vi "Main.vi"(11 "Module Admin":refnum<class "Delacor_lib_QMH_Cloneable Module Admin.lvclass">) -> ()   [LabVIEW 2019, in "Adquisicion2.lvlib"]
doc: "This template is based off of the Queued Message Handler design pattern and the Queued Message Handler project template that ships with LabVIEW.\n\nThe main difference is that the queue is private to this module and communication between modules is performed via Broadcast and Request events.\n\nRequest events are wrapped in public API methods and are handled in the Event Handling Loop (EHL) of this VI. Any module can register for Broadcast events sent by this module. The EHL generates messages based on user interface actions.\n\nThe Message Handling Loop (MHL) processes messages generated by the EHL, or by other messages. The messages are string values, so new messages can be added easily to the Message Cases case structure in the MHL. Each message cluster can also provide an optional value for Message Data, which is a variant that can be converted to whatever message-specific data is required.\n_____\nBased on Delacor QMH Project Template 5.0.0.82."
uses:
  Adquisicion2.lvlib
  <vilib>/Delacor/Delacor QMH/Libraries/Cloneable Module Admin_class/Delacor_lib_QMH_Cloneable Module Admin.lvclass
  C:/Program Files/National Instruments/LabVIEW 2019/vi.lib/Delacor/Delacor QMH/Libraries/Module Admin_class/Delacor_lib_QMH_Module Admin.lvclass
  Module Data--cluster.ctl
  <vilib>/Delacor/Delacor QMH/Libraries/Message Queue_class/Delacor_lib_QMH_Message Queue.lvclass/Delacor_lib_QMH_Message Queue.ctl
  <vilib>/Delacor/Delacor QMH/Libraries/Cloneable Module Admin_class/Delacor_lib_QMH_Cloneable Module Admin.lvclass/Delacor_lib_QMH_Cloneable Module Admin.ctl
  Stop Argument--cluster.ctl
  <vilib>/Delacor/Delacor QMH/Libraries/Module Admin_class/Delacor_lib_QMH_Module Admin.lvclass/Delacor_lib_QMH_Module Admin.ctl
  <vilib>/Utility/miscctls.llb/LVPointTypeDef.ctl
  <vilib>/Delacor/Delacor QMH/Libraries/Message Queue_class/Delacor_lib_QMH_Enqueue Message (Single).vi
  <vilib>/Delacor/Delacor QMH/Libraries/Cloneable Module Admin_class/Delacor_lib_QMH_Get Module ID.vi
  <vilib>/Delacor/Delacor QMH/Libraries/Module Admin_class/Delacor_lib_QMH_Get External Launch.vi
  <vilib>/Utility/error.llb/Error Cluster From Error Code.vi
  <vilib>/ErrorRing/Error Ring.xnode
  <vilib>/Delacor/Delacor QMH/Libraries/Message Queue_class/Delacor_lib_QMH_Message Queue.lvclass
panel:
  in  "Simulate MHL Error":bool
  in  "Simulate EHL Error":bool
  out "error out":errorcluster
  out "Status":string
  # "Other QMH Modules communicate with this Module via its Public API (wrappers for its Request Events).\n\nThis Module communicates with other Modules via its Broadcast Events.\nAny module that wants to get these messages, just registers for this module's Broadcast events."
  # "This template is for the Delacor Modified Queued Message Handler design pattern.\n\nSee the block diagram for more information on how to use this template."
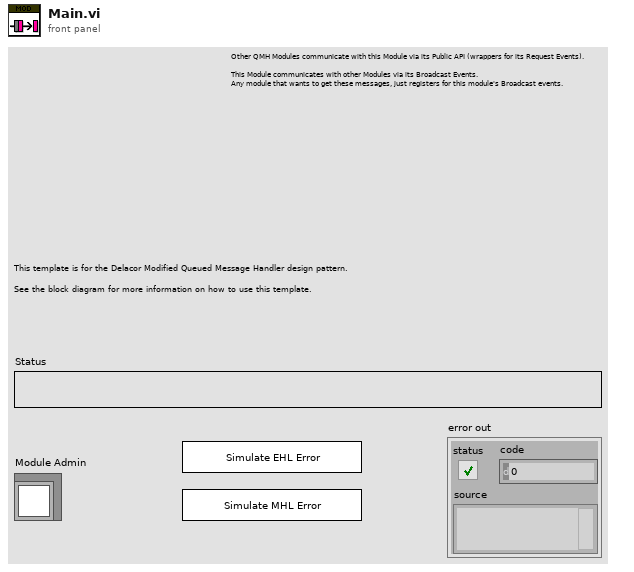
[diagram p1: front panel]
types:
  T1 = typedef "Adquisicion2.lvlib/Request Events--cluster.ctl" = cluster{"Stop Module":refnum<user-event>, "Show Panel":refnum<user-event>, "Hide Panel":refnum<user-event>, "Show Diagram":refnum<user-event>, "Get Module Execution Status":refnum<user-event>}
  T2 = typedef "Adquisicion2.lvlib/Module Data--cluster.ctl" = cluster{"Status":string}
  T3 = enum32{"invalid lock state", "Not Locked", "Locked (No Password)", "Password-protected"}
  T4 = typedef "Adquisicion2.lvlib/Stop Argument--cluster.ctl" = cluster{"Module ID":i32, "Origin":string, "Exit via Stop Module Req?":bool, "Wait for Module to stop?":bool}
  T5 = typedef "LVPointTypeDef.ctl" = cluster{"Horizontal":i16, "Vertical":i16}
  T6 = enum32{"Invalid", "Standard", "Closed", "Hidden", "Minimized", "Maximized"}
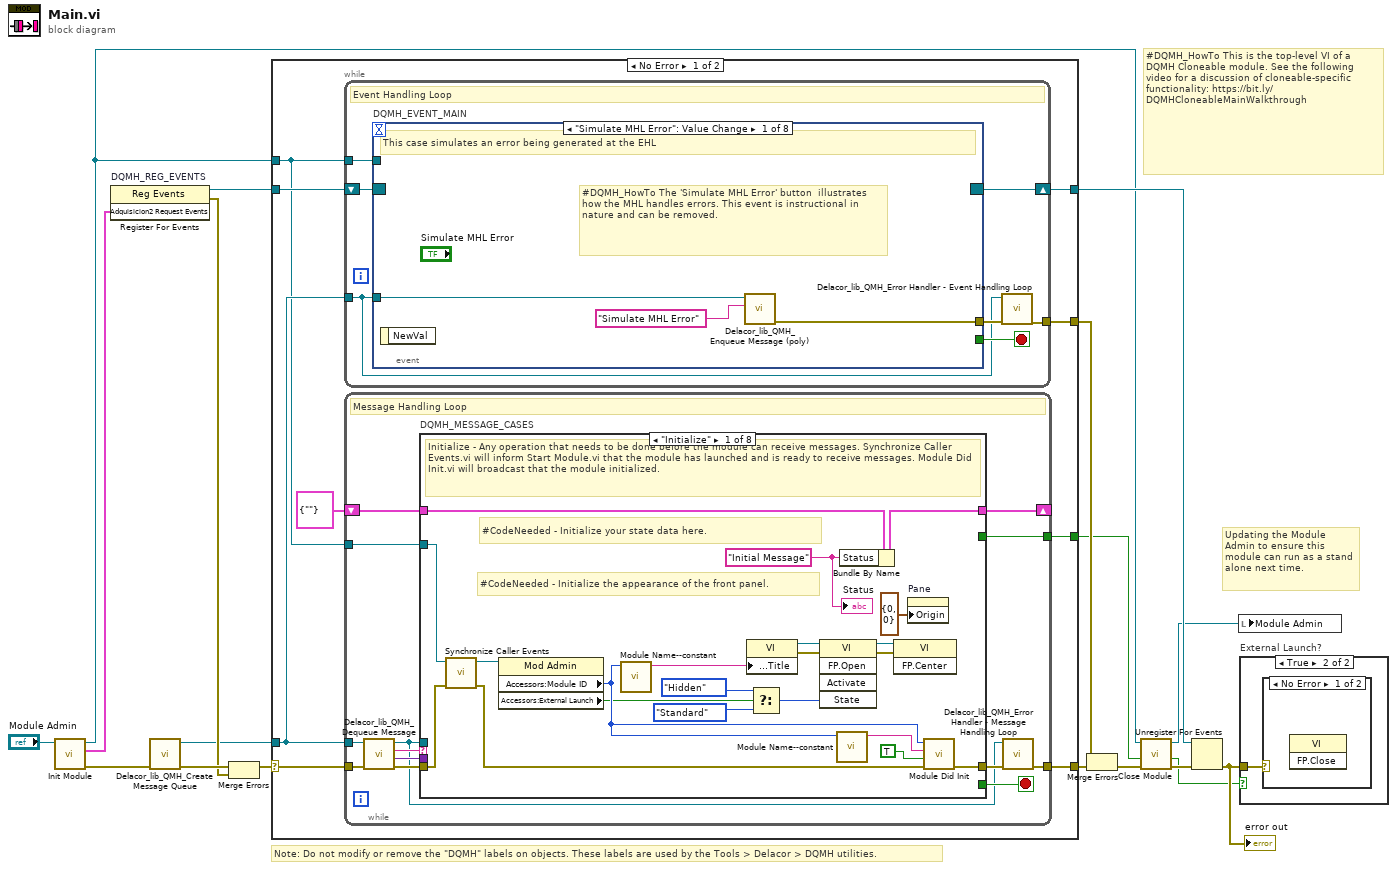
[diagram p0: block diagram]
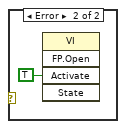
[diagram p3: hidden frame]
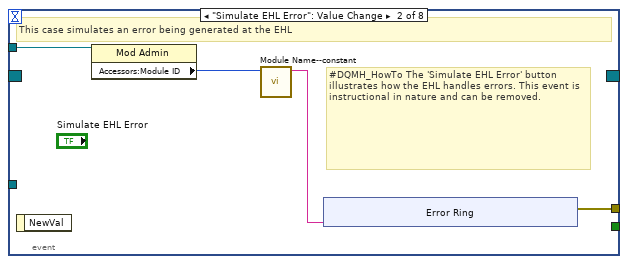
[diagram p4: hidden frame]
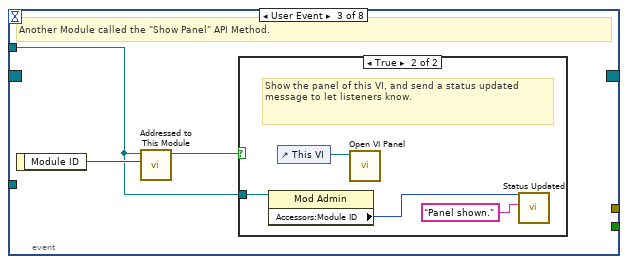
[diagram p5: hidden frame]
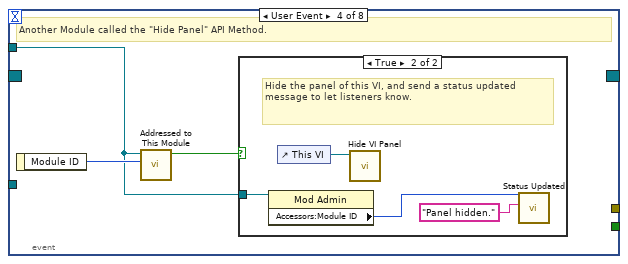
[diagram p7: hidden frame]
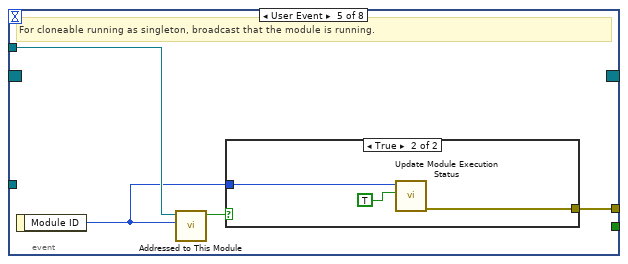
[diagram p9: hidden frame]
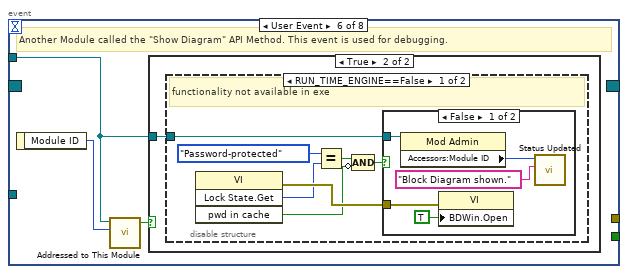
[diagram p11: hidden frame]
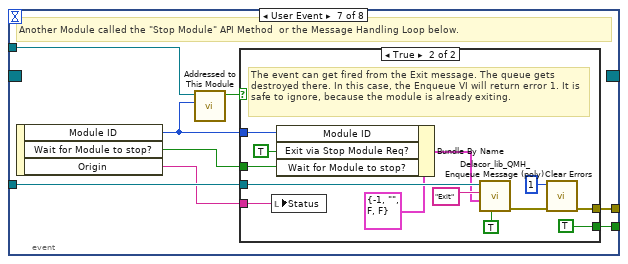
[diagram p15: hidden frame]
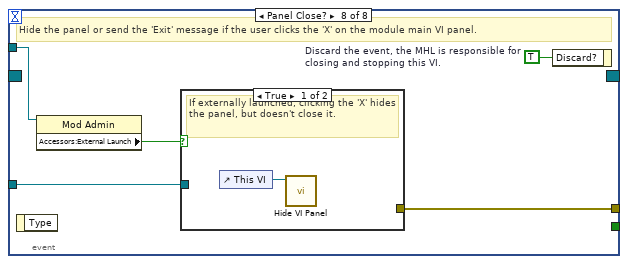
[diagram p17: hidden frame]
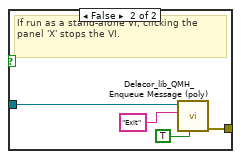
[diagram p18: hidden frame]
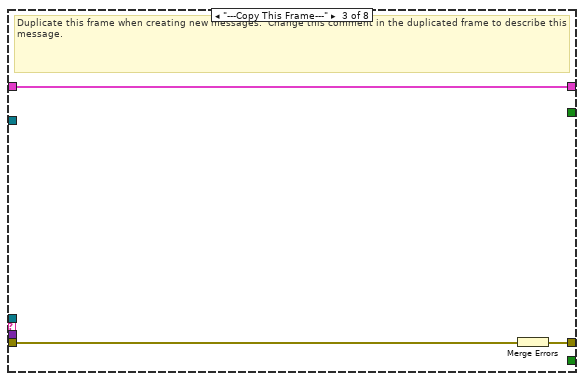
[diagram p20: hidden frame]
diagram:
  # "#DQMH_HowTo This is the top-level VI of a DQMH Cloneable module. See the following video for a discussion of cloneable-specific functionality: https://bit.ly/DQMHCloneableMainWalkthrough"
  # "Note: Do not modify or remove the \"DQMH\" labels on objects. These labels are used by the Tools > Delacor > DQMH utilities."
  # "Updating the Module Admin to ensure this module can run as a stand alone next time."
  n1 = call "Init Module.vi"("Cloneable Module Admin in"="Module Admin") -> ("error out"=w15:errorcluster, "Adquisicion2 Request Events"=w7:T1, "Cloneable Module Admin out"=w4:refnum<class "Delacor_lib_QMH_Cloneable Module Admin.lvclass">)  [unwired: 8 in]
  n2 = register-events "DQMH_REG_EVENTS"(w7) -> (reference out=w8:refnum<event-registration>, error out=w10:errorcluster)  [unwired: 2 in]
  n3 = call <vilib>:"Delacor_lib_QMH_Create Message Queue.vi"("error in (no error)"=w15) -> ("error out"=w12:errorcluster, "Message Queue"=w6:refnum<class "Delacor_lib_QMH_Message Queue.lvclass">)  [unwired: 9 in]
  n4 = Merge Errors(w12, w10) -> (w11:errorcluster)
  n5 = case shown="No Error" w11 {
    selector: w11 -> [w25 w224]
    tunnel: [w27 w223] -> w16
    tunnel: [w24 w231] -> w9
    tunnel: w8 -> [w22 w231]
    tunnel: w6 -> [w21 w222]
    tunnel: [w26 _] -> w17
    tunnel: w4 -> [w20 w227]
    tunnel: [w19 _] -> w2
    frame No Error {
      n6 = while {
        tunnel: w21 -> [w28]
        shift-right: [w31] -> w24
        shift-left: w22 -> [w32]
        tunnel: [w33] -> w26
        tunnel: w20 -> [w29]
        stop <- w30 stop-if-true
        # "Event Handling Loop"
        n7 = event "DQMH_EVENT_MAIN" shown="[0] \"Simulate MHL Error\": Value Change" {
          selector: w32 -> [_ _ _ _ _ _ _ _]
          dyn-events: [_ _ _ _ _ _ _ _] -> w31
          timeout: _ -> [_ _ _ _ _ _ _ _]
          tunnel: [_ _ _ _ _ _ w89 _] -> w30
          tunnel: w28 -> [w36 _ _ _ _ _ w92 w108]
          tunnel: [w37 w41 _ _ w66 _ w93 w111] -> w34
          tunnel: w29 -> [_ w40 w49 w56 w64 w70 w91 w109]
          event "Simulate MHL Error": Value Change {
            # "#DQMH_HowTo The 'Simulate MHL Error' button  illustrates how the MHL handles errors. This event is instructional in nature and can be removed."
            # "This case simulates an error being generated at the EHL"
            n8 = event-data() -> ()  [unwired: 1 in, 1 out]
            n9 = call-poly <vilib>:"Delacor_lib_QMH_Enqueue Message (poly).vi"("Message"="Simulate MHL Error", "Message Queue in"=w36) -> ("error out"=w37:errorcluster)  [unwired: 8 in, 1 out]
          }
          event "Simulate EHL Error": Value Change {
            # "#DQMH_HowTo The 'Simulate EHL Error' button  illustrates how the EHL handles errors. This event is instructional in nature and can be removed."
            # "This case simulates an error being generated at the EHL"
            n10 = event-data() -> ()  [unwired: 1 in, 1 out]
            n11 = property class="Mod Admin"(reference=w40) -> ("Accessors:Module ID"=w39:i32)  [unwired: 1 in, 2 out]
            n12 = call "Module Name--constant.vi"("Module ID"=w39) -> ("Module Name"=w38:string)  [unwired: 10 in]
            n13 = xnode "Error Ring"("parameter 0"=w38) -> ("error out"=w41:errorcluster)
          }
          event User Event {
            # "Another Module called the \"Show Panel\" API Method."
            n14 = event-data() -> ("Module ID"=w50:i32)  [unwired: 1 in]
            n15 = call "Addressed to This Module.vi"("Module ID from Argument"=w50, "Module Admin"=w49) -> ("Addressed to this instance?"=w51:bool)  [unwired: 8 in, 1 out]
            n16 = case shown="True" w51 {
              tunnel: w49 -> [_ w53]
              frame False {
              }
              frame True {
                # "Show the panel of this VI, and send a status updated message to let listeners know."
                n17 = property class="Mod Admin"(reference=w53) -> ("Accessors:Module ID"=w52:i32)  [unwired: 1 in, 2 out]
                n18 = control-ref of="This VI"() -> (w55:refnum<vi>)
                n19 = call "Open VI Panel.vi"("VI"=w55) -> ()  [unwired: 10 in, 1 out]
                n20 = call "Status Updated.vi"("Status"="Panel shown." ("format string"), "Module ID"=w52) -> ()  [unwired: 9 in, 1 out]
              }
            }
          }
          event User Event {
            # "Another Module called the \"Hide Panel\" API Method."
            n21 = event-data() -> ("Module ID"=w57:i32)  [unwired: 1 in]
            n22 = call "Addressed to This Module.vi"("Module ID from Argument"=w57, "Module Admin"=w56) -> ("Addressed to this instance?"=w58:bool)  [unwired: 8 in, 1 out]
            n23 = case shown="True" w58 {
              tunnel: w56 -> [_ w60]
              frame False {
              }
              frame True {
                # "Hide the panel of this VI, and send a status updated message to let listeners know."
                n24 = property class="Mod Admin"(reference=w60) -> ("Accessors:Module ID"=w59:i32)  [unwired: 1 in, 2 out]
                n25 = control-ref of="This VI"() -> (w62:refnum<vi>)
                n26 = call "Hide VI Panel.vi"("VI"=w62) -> ()  [unwired: 10 in, 1 out]
                n27 = call "Status Updated.vi"("Status"="Panel hidden." ("format string"), "Module ID"=w59) -> ()  [unwired: 9 in, 1 out]
              }
            }
          }
          event User Event {
            # "For cloneable running as singleton, broadcast that the module is running."
            n28 = event-data() -> ("Module ID"=w63:i32)  [unwired: 1 in]
            n29 = call "Addressed to This Module.vi"("Module ID from Argument"=w63, "Module Admin"=w64) -> ("Addressed to this instance?"=w65:bool)  [unwired: 8 in, 1 out]
            n30 = case shown="True" w65 {
              tunnel: [_ w69] -> w66
              tunnel: w63 -> [_ w68]
              frame False {
              }
              frame True {
                n31 = call "Update Module Execution Status.vi"("Running?"=TRUE, "Module ID"=w68) -> ("error out"=w69:errorcluster)  [unwired: 9 in]
              }
            }
          }
          event User Event {
            # "Another Module called the \"Show Diagram\" API Method. This event is used for debugging."
            n32 = event-data() -> ("Module ID"=w71:i32)  [unwired: 1 in]
            n33 = call "Addressed to This Module.vi"("Module ID from Argument"=w71, "Module Admin"=w70) -> ("Addressed to this instance?"=w72:bool)  [unwired: 8 in, 1 out]
            n34 = case shown="True" w72 {
              tunnel: w70 -> [_ w73]
              frame False {
              }
              frame True {
                n35 = disable-structure shown="RUN_TIME_ENGINE==False" {
                  disable-tunnel: w73 -> [w74 _]
                  frame condition #0 (active) {
                    # "functionality not available in exe"
                    n36 = invoke class="VI" method="Lock State.Get"() -> (error out=w80:errorcluster, "Get Lock State"=w79:T3, "pwd in cache"=w76:bool)  [unwired: 4 in, 1 out]
                    n37 = Equal?(x=T3."Password-protected", y=w79) -> (x = y?=w77:bool)
                    n38 = Compound Arithmetic op=AND(w77, invert w76) -> (w75:bool)
                    n39 = case shown="False" w75 {
                      tunnel: w80 -> [w85 _]
                      tunnel: w74 -> [w82 _]
                      frame False {
                        n40 = property class="Mod Admin"(reference=w82) -> ("Accessors:Module ID"=w81:i32)  [unwired: 1 in, 2 out]
                        n41 = property class="VI"(error in=w85, "BDWin.Open"=TRUE ("Block Diagram Window:Open")) -> ()  [unwired: 1 in, 2 out]
                        n42 = call "Status Updated.vi"("Status"="Block Diagram shown." ("format string"), "Module ID"=w81) -> ()  [unwired: 9 in, 1 out]
                      }
                      frame True {
                        # "Password-protected VI, and the password is not in the cache. Do not show the diagram."
                      }
                    }
                  }
                  frame condition #1 {
                  }
                }
              }
            }
          }
          event User Event {
            # "Another Module called the \"Stop Module\" API Method  or the Message Handling Loop below."
            n43 = event-data() -> ("Module ID"=w87:i32, "Wait for Module to stop?"=w88:bool, "Origin"=w86:string)  [unwired: 1 in]
            n44 = call "Addressed to This Module.vi"("Module ID from Argument"=w87, "Module Admin"=w91) -> ("Addressed to this instance?"=w90:bool)  [unwired: 8 in, 1 out]
            n45 = case shown="True" w90 {
              tunnel: [_ w105] -> w93
              tunnel: w92 -> [_ w101]
              tunnel: [_ TRUE] -> w89
              tunnel: w88 -> [_ w96]
              tunnel: w87 -> [_ w98]
              tunnel: w86 -> [_ w94]
              frame False {
              }
              frame True {
                # "The event can get fired from the Exit message. The queue gets destroyed there. In this case, the Enqueue VI will return error 1. It is safe to ignore, because the module is already exiting."
                n46 = local write "Status"(w94) -> ()
                n47 = Bundle By Name(cluster=T4 {"Module ID"=-1, "Origin"="", "Exit via Stop Module Req?"=FALSE, "Wait for Module to stop?"=FALSE} ("Stop Argument"), "Module ID"=w98, "Exit via Stop Module Req?"=TRUE, "Wait for Module to stop?"=w96) -> (w95:T4)
                n48 = call-poly <vilib>:"Delacor_lib_QMH_Enqueue Message (poly).vi"("Priority Message? (F)"=TRUE, "Message Data"=w95, "Message"="Exit", "Message Queue in"=w101) -> ("error out"=w106:errorcluster)  [unwired: 6 in, 1 out]
                n49 = call <vilib>:"Clear Errors.vi"("error in (no error)"=w106, "specific error code to clear (0: all)"=1) -> ("error out"=w105:errorcluster)  [unwired: 4 in, 1 out]
              }
            }
          }
          event Panel Close? {
            w110 = TRUE  # Discard the event, the MHL is responsible for closing and stopping this VI.
            # "Hide the panel or send the 'Exit' message if the user clicks the 'X' on the module main VI panel."
            n50 = event-data() -> ()  [unwired: 1 in, 1 out]
            n51 = property class="Mod Admin"(reference=w109) -> ("Accessors:External Launch"=w107:bool)  [unwired: 1 in, 2 out]
            n52 = case shown="True" w107 {
              tunnel: w108 -> [_ w115]
              tunnel: [_ w116] -> w111
              frame True {
                # "If externally launched, clicking the 'X' hides the panel, but doesn't close it."
                n53 = control-ref of="This VI"() -> (w112:refnum<vi>)
                n54 = call "Hide VI Panel.vi"("VI"=w112) -> ()  [unwired: 10 in, 1 out]
              }
              frame False {
                # "If run as a stand-alone VI, clicking the panel 'X' stops the VI."
                n55 = call-poly <vilib>:"Delacor_lib_QMH_Enqueue Message (poly).vi"("Priority Message? (F)"=TRUE, "Message"="Exit", "Message Queue in"=w115) -> ("error out"=w116:errorcluster)  [unwired: 7 in, 1 out]
              }
            }
            n56 = event-data("Discard?"=w110) -> ()  [unwired: 1 in, 1 out]
          }
        }
        n57 = call-dynamic "Delacor_lib_QMH_Error Handler - Event Handling Loop.vi"("error in (no error)"=w34, "Message Queue in"=w28) -> ("dup error in"=w33:errorcluster)  [unwired: 8 in, 1 out]
      }
      n58 = while {
        tunnel: w21 -> [w120]
        shift-right: [w124] -> _
        shift-left: T2 {"Status"=""} ("Data Cluster") -> [w125]
        tunnel: w25 -> [w128]
        tunnel: [w126] -> w27
        tunnel: w20 -> [w118]
        tunnel: [w117] -> w19
        stop <- w123 stop-if-true
        # "Message Handling Loop"
        n59 = call-dynamic "Delacor_lib_QMH_Dequeue Message.vi"("error in (no error)"=w128, "Message Queue in"=w120) -> ("error out"=w127:errorcluster, "Message Data"=w121:variant, "Message"=w122:string, "Message Queue out"=w119:refnum<class "Delacor_lib_QMH_Message Queue.lvclass">)  [unwired: 6 in]
        n60 = case "DQMH_MESSAGE_CASES" shown="\"Initialize\"" w122 {
          selector: w122 -> [_ _ _ _ _ _ _ w209]
          tunnel: w119 -> [_ _ _ _ w160 _ w199 _]
          tunnel: w127 -> [w148 w152 w155 w157 w169 w182 w205 w211]
          tunnel: [w146 w152 w154 w157 w165 w181 w202 w212] -> w129
          tunnel: w125 -> [w139 w151 w153 w156 w164 w179 w198 w210]
          tunnel: [w138 w151 w153 w156 w164 w179 w198 w210] -> w124
          tunnel: [_ _ _ _ _ _ w197 _] -> w123
          tunnel: w121 -> [_ _ _ _ w163 _ w195 _]
          tunnel: w118 -> [w133 _ _ _ w162 w177 w191 w207]
          tunnel: [_ _ _ _ _ _ w193 _] -> w117
          frame "Initialize" {
            w130 = "Initial Message" ("Initial Message")
            # "#CodeNeeded - Initialize the appearance of the front panel."
            # "#CodeNeeded - Initialize your state data here."
            # "Initialize - Any operation that needs to be done before the module can receive messages. Synchronize Caller Events.vi will inform Start Module.vi that the module has launched and is ready to receive messages. Module Did Init.vi will broadcast that the module initialized."
            n61 = call "Synchronize Caller Events.vi"("error in (no error)"=w148, "Module Admin"=w133) -> ("error out"=w147:errorcluster, "Module Admin out"=w132:refnum<class "Delacor_lib_QMH_Cloneable Module Admin.lvclass">)  [unwired: 8 in]
            n62 = property class="Mod Admin"(reference=w132) -> ("Accessors:Module ID"=w135:i32, "Accessors:External Launch"=w134:bool)  [unwired: 1 in, 2 out]
            n63 = call "Module Name--constant.vi"("Module ID"=w135) -> ("Module Name"=w143:string)  [unwired: 10 in]
            n64 = property class="VI"("Front Panel.Title"=w143) -> (reference out=w145:refnum<vi>, error out=w150:errorcluster)  [unwired: 2 in]
            n65 = Select(t=T6."Hidden" ("State"), s=w134, f=T6."Standard" ("State")) -> (s? t:f=w140:T6)
            n66 = invoke class="VI" method="FP.Open"(reference=w145, error in=w150, "State"=w140) -> (reference out=w144:refnum<vi>, error out=w149:errorcluster)  [unwired: 2 in, 3 out]
            n67 = call "Module Name--constant.vi"("Module ID"=w135) -> ("Module Name"=w136:string)  [unwired: 10 in]
            n68 = Bundle By Name(cluster=w139, "Status"=w130) -> (w138:T2)
            n69 = invoke class="VI" method="FP.Center"(reference=w144, error in=w149) -> ()  [unwired: 1 in, 3 out]
            n70 = property on="Pane" class="Pane"("Origin"=T5 {"Horizontal"=0, "Vertical"=0}) -> ()  [unwired: 2 in, 2 out]
            n71 = call "Module Did Init.vi"("error in (no error)"=w147, "Initialized?"=TRUE, "Origin"=w136, "Module ID"=w135) -> ("error out"=w146:errorcluster)  [unwired: 7 in]
            "Status" <- w130
          }
          frame "--- Module Specific ---" {
            # "Separator -- The following cases handle messages specific to this Module."
          }
          frame "---Copy This Frame---" {
            # "Duplicate this frame when creating new messages.  Change this comment in the duplicated frame to describe this message."
            n72 = Merge Errors(w155) -> (w154:errorcluster)
          }
          frame "--- Exit and Error Handling---" {
            # "Separator - the following cases handle errors and exit messages."
          }
          frame "Error" {
            # "#CodeRecommended - If you ever change the name of this \"Error\" message, you'll need to update the name in the Check Loop Error.vi as well."
            # "#CodeRecommended - If the module is running in standalone mode (External Launch = FALSE), this code will pop up an error dialog and call the 'Exit' message if an error occurs. Add more fine-grained error handling here."
            # "Error - Check the error message data and respond accordingly. This message is sent by the \"Error Handler\" VIs at the end of each loop in this application."
            n73 = property class="Mod Admin"(reference=w162) -> ("Accessors:External Launch"=w161:bool, "Accessors:Module ID"=w158:i32)  [unwired: 1 in, 2 out]
            n74 = Variant To Data(error in=w169, type=errorcluster {"status"=FALSE, "code"=0, "source"=""} ("error constant"), Variant=w163) -> (data=w170:errorcluster, error out=w167:errorcluster)
            n75 = call "Module Name--constant.vi"("Module ID"=w158) -> ("Module Name"=w159:string)  [unwired: 10 in]
            n76 = call "Error Reported.vi"("Additional Information"=w159, "Error"=w170, "Module ID"=w158) -> ()  [unwired: 8 in, 1 out]
            n77 = case shown="False" w161 {
              tunnel: [w175 _] -> w166
              tunnel: w160 -> [w173 _]
              tunnel: w170 -> [w174 _]
              frame False {
                # "If the module is running standalone, then pop up an error dialog and call the \"Exit\" message."
                n78 = call <vilib>:"Simple Error Handler.vi"("error in (no error)"=w174) -> ()  [unwired: 4 in, 5 out]
                n79 = call-poly <vilib>:"Delacor_lib_QMH_Enqueue Message (poly).vi"("Priority Message? (F)"=TRUE, "Message"="Exit", "Message Queue in"=w173) -> ("error out"=w175:errorcluster)  [unwired: 7 in, 1 out]
              }
              frame True {
                # "If the module was launched externally, calling the Error Reported broadcast VI is the only action performed by the \"Error\" message. The module's caller can then process the error appropriately."
              }
            }
            n80 = Merge Errors(w167, w166) -> (w165:errorcluster)
            n81 = local write "error out"(w165) -> ()
          }
          frame "Simulate MHL Error" {
            # "#DQMH_HowTo The 'Simulate MHL Error' button  illustrates how the MHL handles errors. This event is instructional in nature and can be removed."
            # "Simulate an error occurring at the MHL"
            n82 = property class="Mod Admin"(reference=w177) -> ("Accessors:Module ID"=w178:i32)  [unwired: 1 in, 2 out]
            n83 = call "Module Name--constant.vi"("Module ID"=w178) -> ("Module Name"=w176:string)  [unwired: 10 in]
            n84 = xnode "Error Ring"("parameter 0"=w176) -> ("error out"=w180:errorcluster)
            n85 = Merge Errors(w182, w180) -> (w181:errorcluster)
          }
          frame "Exit" {
            w196 = 91  # 91: not all Exit messages will have an argument
            w197 = TRUE  # Stop the VI
            # "Release the message queue reference"
            # "#CodeNeeded - Add any required cleanup code here."
            # "Exit - Exit the application."
            n86 = Variant To Data(error in=w205, type=T4 {"Module ID"=-1, "Origin"="", "Exit via Stop Module Req?"=FALSE, "Wait for Module to stop?"=FALSE} ("Stop Argument"), Variant=w195) -> (data=w192:T4, error out=w200:errorcluster)
            n87 = call <vilib>:"Clear Errors.vi"("error in (no error)"=w200, "specific error code to clear (0: all)"=w196) -> ("error out"=w204:errorcluster)  [unwired: 4 in, 1 out]
            n88 = control-ref of="This VI"() -> (w190:refnum<vi>)
            n89 = call-dynamic "Delacor_lib_QMH_Release Message Queue.vi"("error in (no error)"=w204, "Message Queue"=w199) -> ("error out"=w203:errorcluster)  [unwired: 9 in]
            n90 = call "Handle Exit.vi"("Stop Argument"=w192, "Module Admin in"=w191, "VI reference"=w190) -> ("error out"=w201:errorcluster, "Wait for Stop?"=w193:bool)  [unwired: 7 in]
            n91 = Merge Errors(w203, w201) -> (w202:errorcluster)
          }
          frame Default {
            # "'Default' case only runs if there is a message that isn't defined in any of the other cases.  Output a programming error."
            n92 = property class="Mod Admin"(reference=w207) -> ("Accessors:Module ID"=w206:i32)  [unwired: 1 in, 2 out]
            n93 = call "Module Name--constant.vi"("Module ID"=w206) -> ("Module Name"=w208:string)  [unwired: 10 in]
            n94 = xnode "Error Ring"("parameter 0"=w209, "parameter 1"=w208) -> ("error out"=w213:errorcluster)
            n95 = Merge Errors(w211, w213) -> (w212:errorcluster)
          }
        }
        n96 = call-dynamic "Delacor_lib_QMH_Error Handler - Message Handling Loop.vi"("error in (no error)"=w129, "Message Queue in"=w119) -> ("dup error in"=w126:errorcluster)  [unwired: 8 in, 1 out]
      }
    }
    frame Error {
      n97 = call "Synchronize Caller Events.vi"("Module Admin"=w227) -> ("Module Admin out"=w226:refnum<class "Delacor_lib_QMH_Cloneable Module Admin.lvclass">)  [unwired: 9 in, 1 out]
      n98 = property class="Mod Admin"(reference=w226) -> ("Accessors:Module ID"=w225:i32)  [unwired: 1 in, 2 out]
      n99 = call-dynamic "Delacor_lib_QMH_Release Message Queue.vi"("error in (no error)"=w224, "Message Queue"=w222) -> ("error out"=w223:errorcluster)  [unwired: 9 in]
      n100 = call "Module Name--constant.vi"("Module ID"=w225) -> ("Module Name"=w230:string)  [unwired: 10 in]
      n101 = Format Into String(format string="An error occurred during initialization. %s is no longer running.", w230) -> (resulting string=w228:string)  [unwired: 2 in, 1 out]
      n102 = call "Error Reported.vi"("Additional Information"=w228, "Error"=w223, "Module ID"=w225) -> ()  [unwired: 8 in, 1 out]
    }
  }
  n103 = Merge Errors(w17, w16) -> (w18:errorcluster)
  n104 = call "Close Module.vi"("error in"=w18, "Wait for stop?"=w2, "Module Admin in"=w4) -> ("error out"=w14:errorcluster, "External Launch"=w1:bool, "Module Admin out"=w3:refnum<class "Delacor_lib_QMH_Cloneable Module Admin.lvclass">)  [unwired: 6 in]
  n105 = Unregister For Events(event registration refnum=w9, error in=w14) -> (error out=w13:errorcluster)
  "error out" <- w13
  n106 = local write "Module Admin"(w3) -> ()
  n107 = case "External Launch?" shown="True" w1 {
    tunnel: w13 -> [_ w232]
    frame False {
    }
    frame True {
      n108 = case shown="No Error" w232 {
        frame No Error {
          n109 = invoke class="VI" method="FP.Close"() -> ()  [unwired: 3 in, 3 out]
        }
        frame Error {
          n110 = invoke class="VI" method="FP.Open"("Activate"=TRUE ("Activate?")) -> ()  [unwired: 4 in, 5 out]
        }
      }
    }
  }
